vi "Cluster.vi"() -> ()   [LabVIEW 2020]
panel:
  out "DATA_ESP32.ADC":dbl[](array[numeric])
  out "output cluster 2":T1
  in  "DO":bool[](array[boolean])
  in  "Selector":u8(knob) scale=0.0..10.0
  in  "CMD HMI":string
  in  "Termocupla":dbl(slide) scale=0.0..100.0
  in  "Boolean":bool
  out "output cluster":T2
  in  "METER":dbl(knob) scale=0.0..60.0
  out "SEND HMI":string
  out "Velocidad":dbl
  out "Pesaje":dbl
  out "Start":bool
  in  "Pesadora de Pescado":T2 {"Velocidad" scale=0.0..60.0}
  # "Cluster"
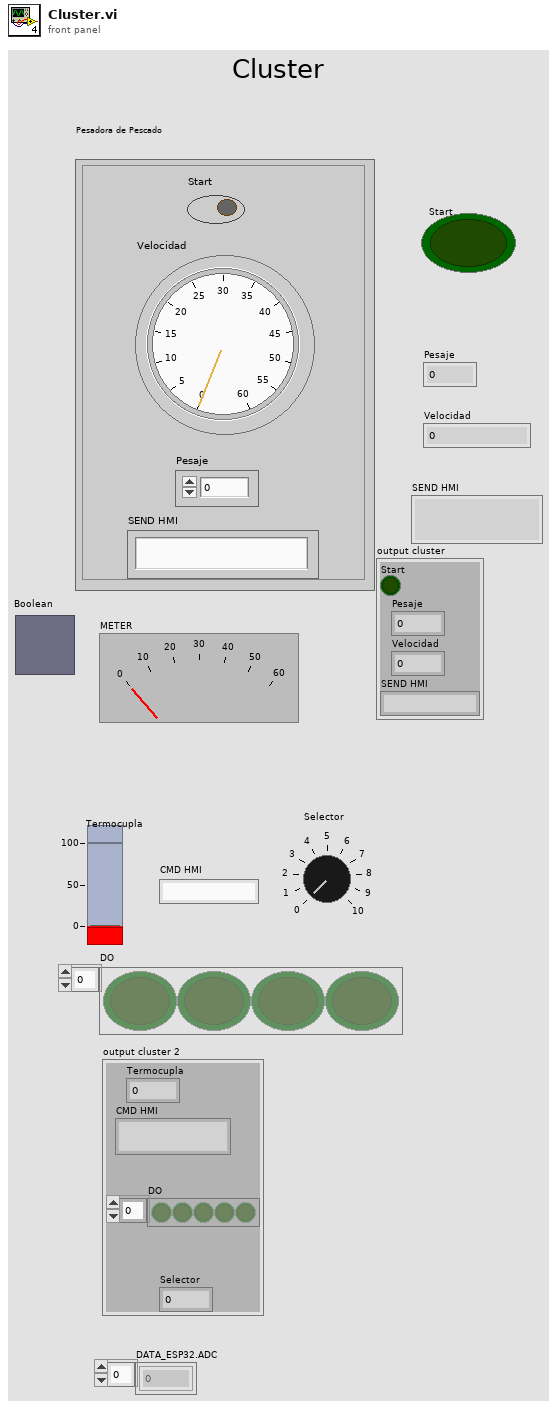
[diagram p1: front panel]
types:
  T1 = cluster{"Termocupla":dbl, "CMD HMI":string, "DO":bool[], "Selector":u8}
  T2 = cluster{"Start":bool, "Pesaje":dbl, "Velocidad":dbl, "SEND HMI":string}
  T3 = cluster{"DATA_ESP32":cluster{"ADC":dbl[], "UART":string, "ON/OFF":bool}, "DATA_PLC":cluster{"Direccion IP":string, "Puerto":i32, "Encoder":i32[], "Variadores":dbl[]}, "DATA_IOT":cluster{"Dominio":string, "Puerto MQTT":i32, "TOKEN":string, "DEVICE":string}, "Warnings":cluster{"Alarmas":bool[]}}
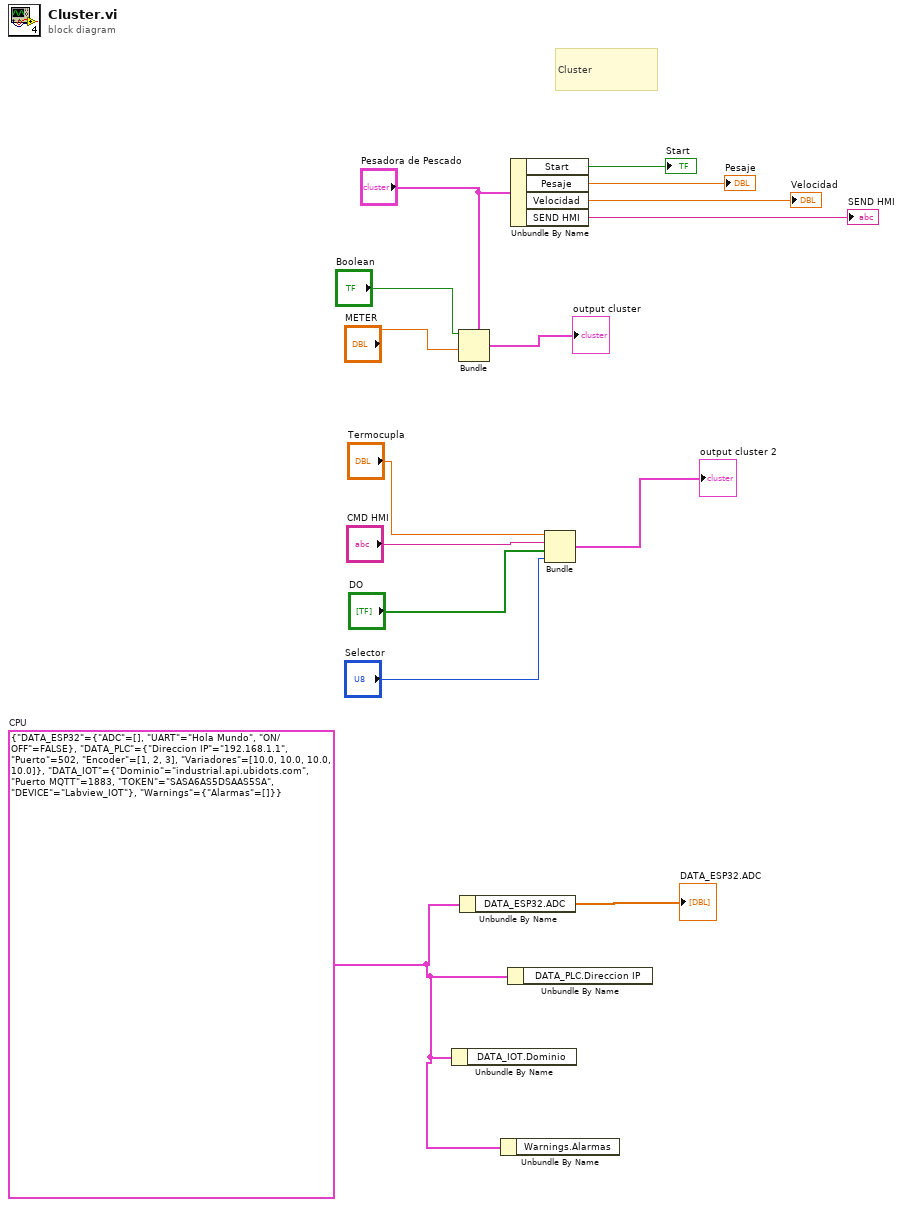
[diagram p0: block diagram]
diagram:
  w1 = T3 {"DATA_ESP32"={"ADC"=[], "UART"="Hola Mundo", "ON/OFF"=FALSE}, "DATA_PLC"={"Direccion IP"="192.168.1.1", "Puerto"=502, "Encoder"=[1, 2, 3], "Variadores"=[10.0, 10.0, 10.0, 10.0]}, "DATA_IOT"={"Dominio"="industrial.api.ubidots.com", "Puerto MQTT"=1883, "TOKEN"="SASA6AS5DSAAS5SA", "DEVICE"="Labview_IOT"}, "Warnings"={"Alarmas"=[]}}  # CPU
  # "Cluster"
  n1 = Unbundle By Name(w1) -> ()  [unwired: 1 out]
  n2 = Bundle(cluster="Pesadora de Pescado", "Start"="Boolean", "Velocidad"="METER") -> (→"output cluster":T2)  [unwired: 2 in]
  n3 = Unbundle By Name(w1) -> ("DATA_ESP32.ADC"=→"DATA_ESP32.ADC":dbl[])
  n4 = Unbundle By Name(w1) -> ()  [unwired: 1 out]
  n5 = Unbundle By Name(w1) -> ()  [unwired: 1 out]
  n6 = Unbundle By Name("Pesadora de Pescado") -> ("Start"=→"Start":bool, "Pesaje"=→"Pesaje":dbl, "Velocidad"=→"Velocidad":dbl, "SEND HMI"=→"SEND HMI":string)
  n7 = Bundle("Termocupla"="Termocupla", "CMD HMI"="CMD HMI", "DO"="DO", "Selector"="Selector") -> (→"output cluster 2":T1)  [unwired: 1 in]
